vi "Parse Groups.vi"(11 "Input":string="???.### 1,1,3\n.??..??...?##. 1,1,3\n?#?#?#?#?#?#?#? 1,3,1,6\n????.#...#... 4,1,1\n????.######..#####. 1,6,5\n?###???????? 3,2,1") -> (2 "Counts":i64[][](array[numeric]), 3 "Groups":refnum<class "Group.lvclass">[](array[class]))   [LabVIEW 2020, in "Group.lvclass"]
uses:
  Group.lvclass
  Helpers/Helpers.lvlib
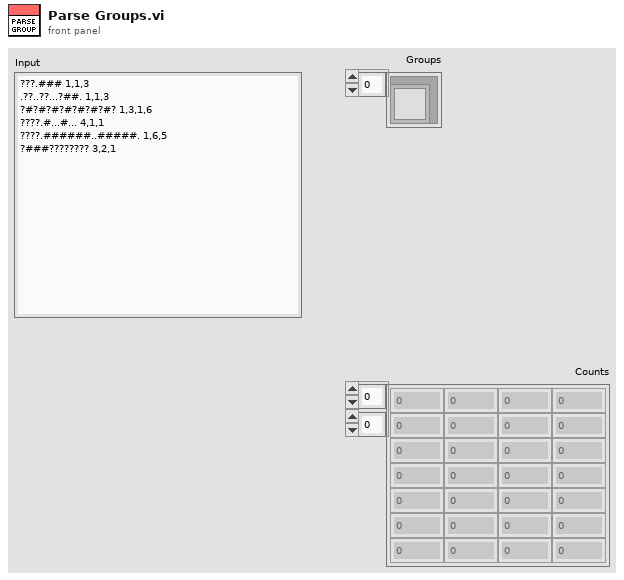
[diagram p1: front panel]
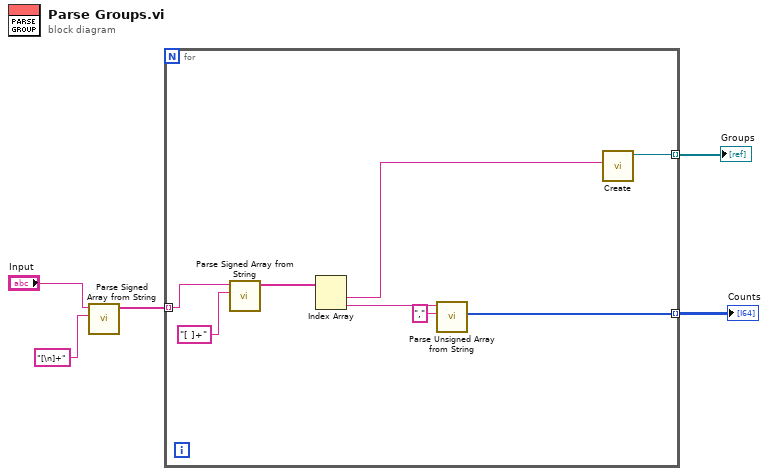
[diagram p0: block diagram]
diagram:
  n1 = call "Parse Signed Array from String.vi"("Delimiter regex"="[\n]+", "Input"="Input") -> ("Parsed Array"=w2:string[])  [unwired: 8 in, 1 out]
  n2 = for {
    tunnel: [w9] -> w5 mode=indexing
    tunnel: w2 -> [w7] mode=indexing
    tunnel: [w6] -> w1 mode=indexing
    n3 = call "Parse Signed Array from String.vi"("Delimiter regex"="[ ]+", "Input"=w7) -> ("Parsed Array"=w12:string[])  [unwired: 8 in, 1 out]
    n4 = Index Array(array=w12) -> (element #1=w8:string, element #2=w11:string)  [unwired: 2 in]
    n5 = call "Parse Unsigned Array from String.vi"("Delimiter regex"=",", "Input"=w11) -> ("Parsed U64 Array"=w6:u64[])  [unwired: 8 in, 1 out]
    n6 = call "Create.vi"("Input"=w8) -> ("Group Out"=w9:refnum<class "Group.lvclass">)  [unwired: 9 in, 1 out]
  }
  "Groups" <- w5
  "Counts" <- w1
